vi "Sysdef.SimpleImport.vi"(7 "Overwrite Existing?":bool=TRUE, 8 "error in (no error)":errorcluster, 10 "SysDef":T1 {"Tree"."Properties"."Type" items=["K_STRING", "K_BOOL", "K_I32", "K_U32", "K_DOUBLE", "K_U64", "K_VARIANT", "K_DEPENDENTFILE", "K_DEPENDENTNODE", "K_DATASOURCENODE", "K_U16", "K_DBLARR", "K_U32ARR", "K_I32ARR", "K_STRINGARR", "K_DICTIONARY", "K_DICTIONARYARR"]}, 11 "NodeID":u64) -> (0 "error out":errorcluster, 3 "NodeID out":u64)   [LabVIEW 2015, in "Import - Export CD Config Utility.lvlib"]
doc: "Uses the NI VeriStand .NET API. to add or edit the Custom Device Hierarchy (Sections, Channels, Waveforms) as well as its Items Properties using the data from the SysDef cluster."
uses:
  Import - Export CD Config Utility.lvlib
  _Types/SysDef.Export.ctl
  _Types/TreeItem.ctl
  _Types/TreeItem.Info.ctl
  <vilib>/NI Veristand/Custom Device API/Custom Device Channel.ctl
  <vilib>/NI Veristand/Custom Device API/Custom Device Channel Type.ctl
  <vilib>/NI Veristand/Custom Device API/Custom Device Waveform.ctl
  <vilib>/NI Veristand/Custom Device API/Custom Device Waveform DataType.ctl
  _Types/TreeItem.Property.ctl
  NationalInstruments.VeriStand.SystemDefinitionAPI
  NationalInstruments.VeriStand.SystemStorage
  <vilib>/NI Veristand/Custom Device API/Custom Device API.lvlib
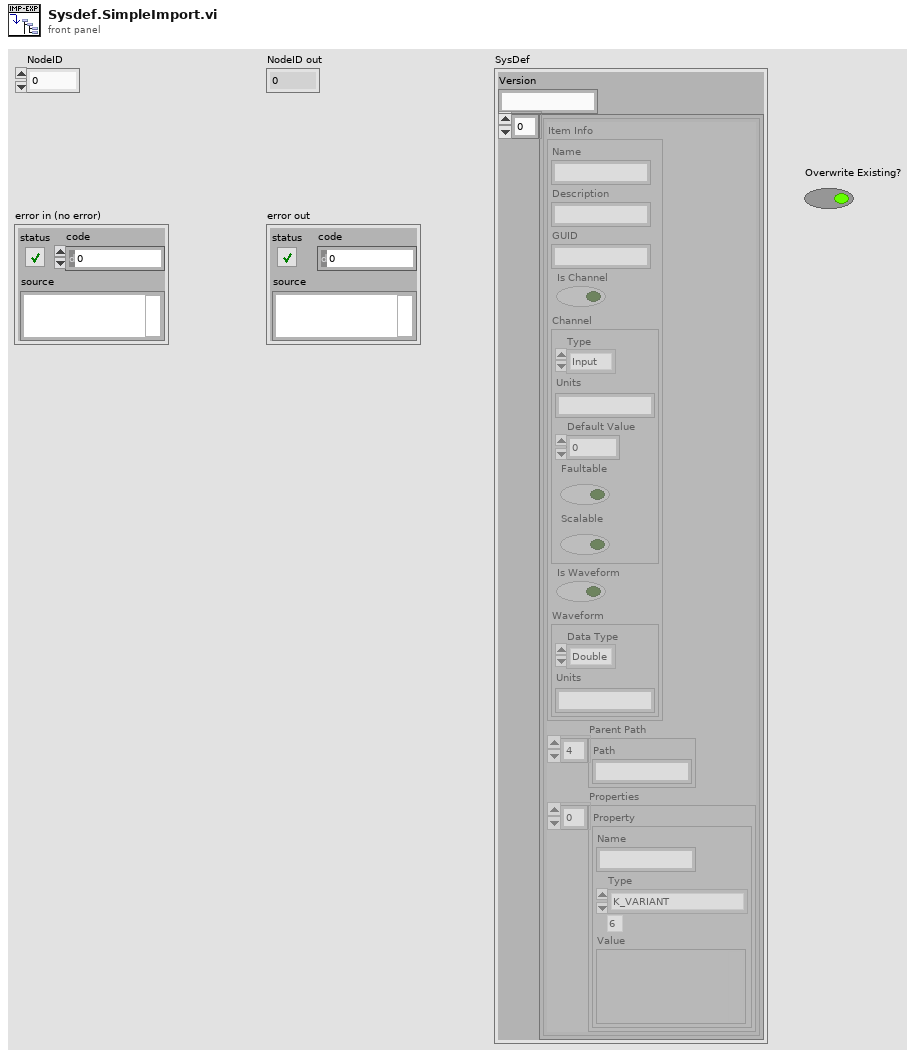
[diagram p1: front panel]
types:
  T1 = typedef "Import - Export CD Config Utility.lvlib/SysDef.Export.ctl" = cluster{"Version":string, "Tree":T2[]}
  T2 = typedef "Import - Export CD Config Utility.lvlib/TreeItem.ctl" = cluster{"Item Info":T3, "Parent Path":string[], "Properties":T8[]}
  T3 = typedef "Import - Export CD Config Utility.lvlib/TreeItem.Info.ctl" = cluster{"Name":string, "Description":string, "GUID":string, "Is Channel":bool, "Channel":T4, "Is Waveform":bool, "Waveform":T6}
  T4 = typedef "Custom Device API.lvlib/Custom Device Channel.ctl" = cluster{"Type":T5, "Units":string, "Default Value":dbl, "Faultable":bool, "Scalable":bool}
  T5 = typedef "Custom Device API.lvlib/Custom Device Channel Type.ctl" = enum16{"Input", "Output"}
  T6 = typedef "Custom Device API.lvlib/Custom Device Waveform.ctl" = cluster{"Data Type":T7, "Units":string}
  T7 = typedef "Custom Device API.lvlib/Custom Device Waveform DataType.ctl" = enum16{"Double", "Complex Double"}
  T8 = typedef "Import - Export CD Config Utility.lvlib/TreeItem.Property.ctl" = cluster{"Name":string, "Type":i32, "Value":variant}
  T9 = typedef "Custom Device API.lvlib/Custom Device Item Ref.ctl" = u64
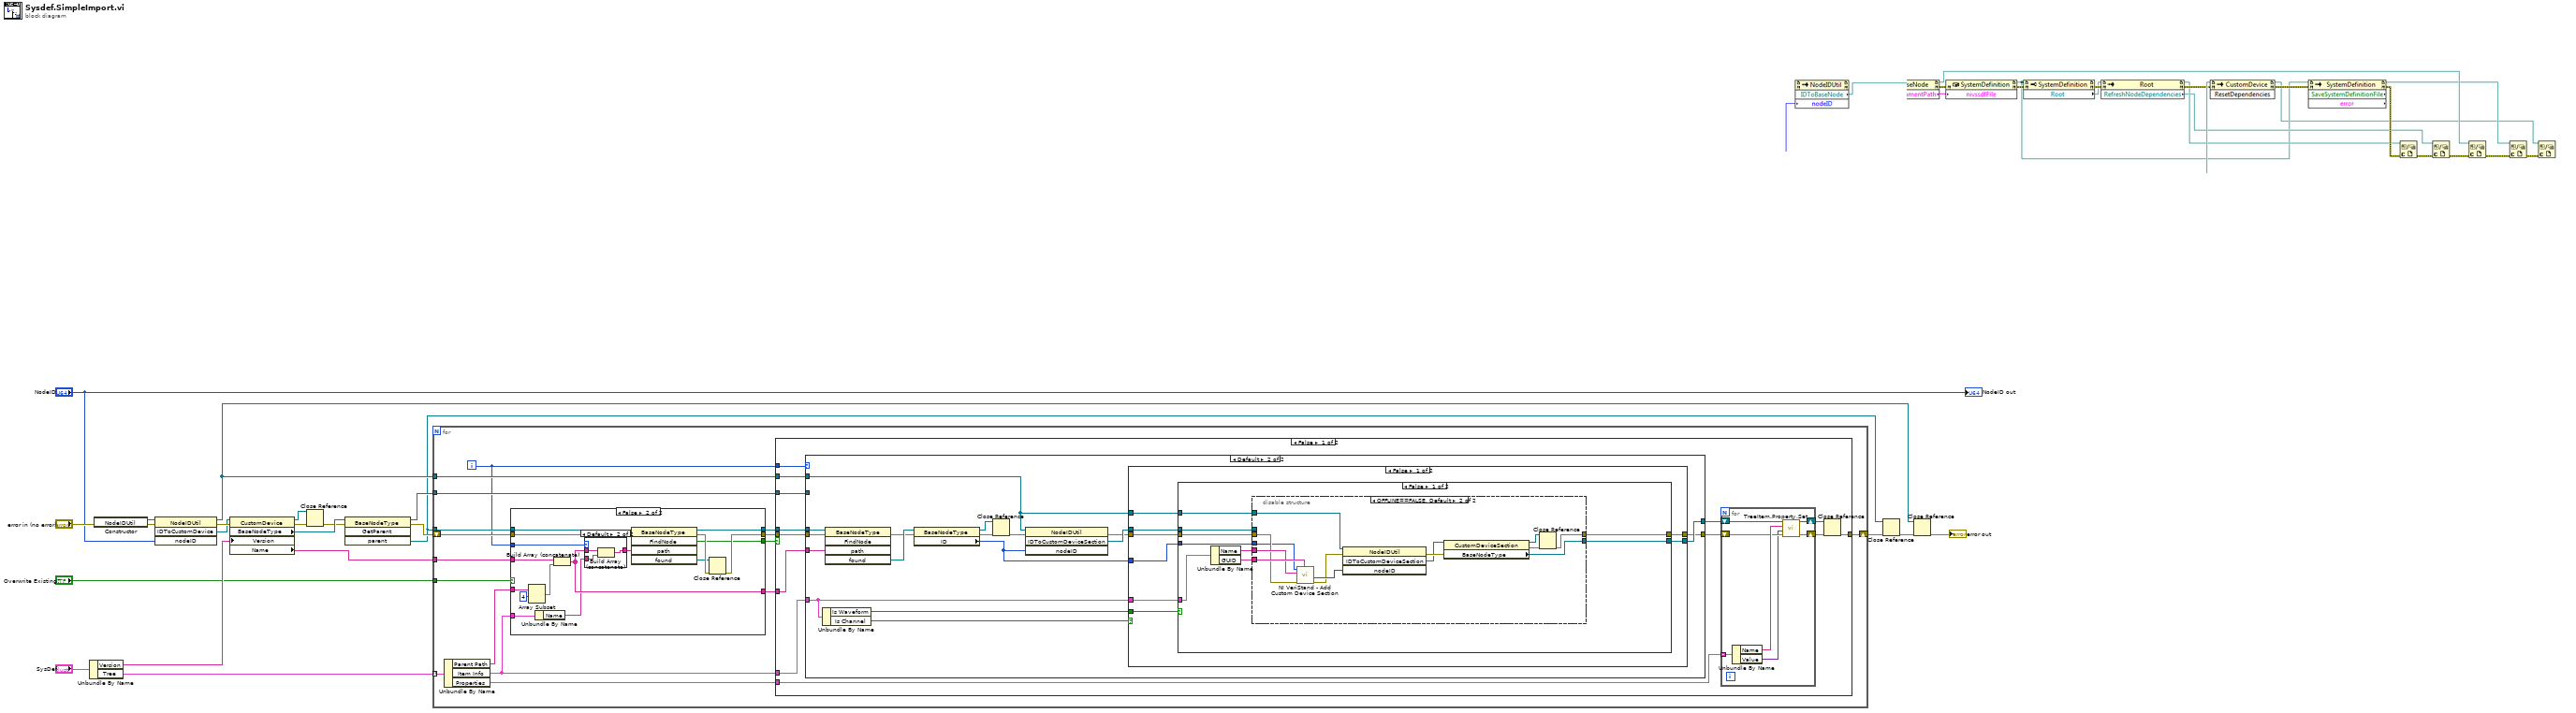
[diagram p0: block diagram]
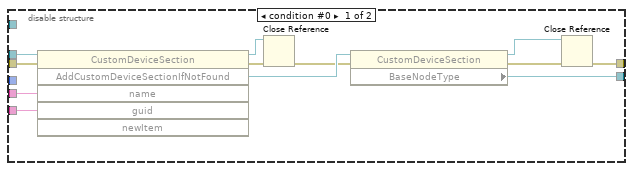
[diagram p3: hidden frame]
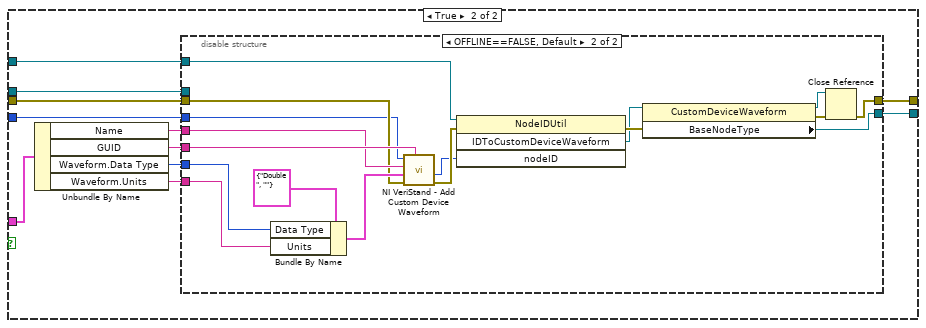
[diagram p4: hidden frame]
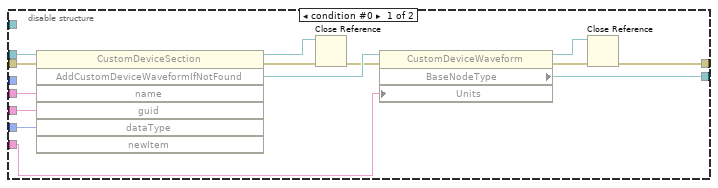
[diagram p5: hidden frame]
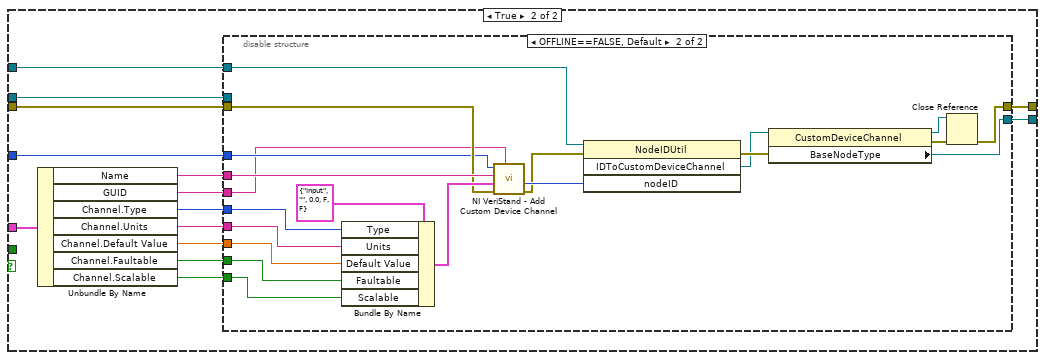
[diagram p6: hidden frame]
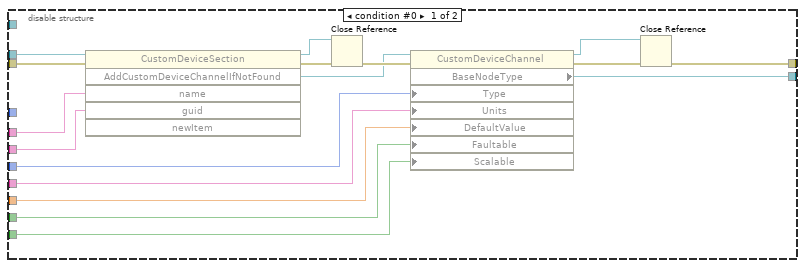
[diagram p7: hidden frame]
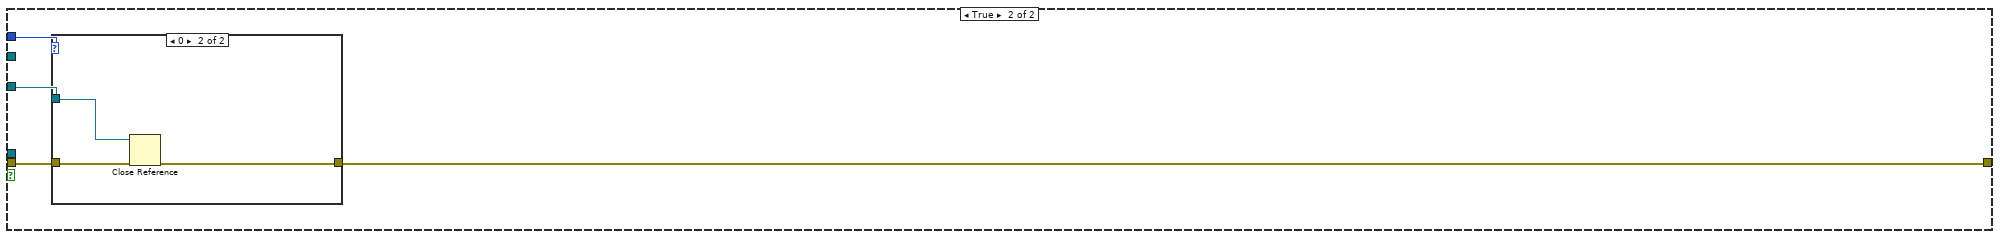
[diagram p8: hidden frame]
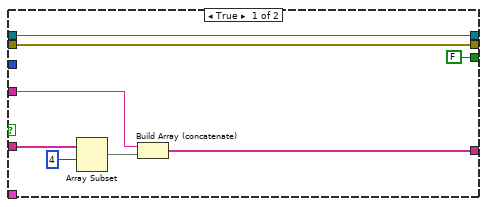
[diagram p10: hidden frame]
diagram:
  n1 = Unbundle By Name("SysDef") -> ("Version"=w20:string, "Tree"=w21:T2[])
  n2 = constructor class="NodeIDUtil"(error in="error in (no error)") -> (reference out=w2:refnum<k24>, error out=w7:errorcluster)  [unwired: 2 in, 1 out]
  n3 = invoke class="NodeIDUtil" method="IDToCustomDevice"(reference=w2, error in=w7, "nodeID"="NodeID") -> (reference out=w13:refnum<k24>, error out=w19:errorcluster, "IDToCustomDevice"=w1:refnum<k24>)  [unwired: 1 in, 1 out]
  n4 = property class="CustomDevice"(reference=w1, error in=w19, "Version"=w20) -> (reference out=w5:refnum<k24>, error out=w4:errorcluster, "BaseNodeType"=w10:refnum<k24>, "Name"=w16:string)
  n5 = Close Reference(reference=w5, error in (no error)=w4) -> (error out=w3:errorcluster)
  n6 = invoke class="BaseNodeType" method="GetParent"(reference=w10, error in=w3) -> (reference out=w17:refnum<k24>, error out=w18:errorcluster, "parent"=w9:refnum<k24>)  [unwired: 2 in, 1 out]
  n7 = for {
    tunnel: w21 -> [w38] mode=indexing
    shift-right: [w35] -> w6
    shift-left: w18 -> [w29]
    tunnel: w17 -> [w34]
    tunnel: w16 -> [w33]
    tunnel: "Overwrite Existing?" -> [w30]
    tunnel: w13 -> [w25]
    tunnel: w9 -> [w24]
    i -> [w23]
    n8 = Unbundle By Name(w38) -> ("Parent Path"=w36:string[], "Item Info"=w31:T3, "Properties"=w37:T8[])
    n9 = case shown="False" w30 {
      tunnel: w36 -> [w227 w243]
      tunnel: w33 -> [w225 w241]
      tunnel: [w224 w239] -> w32
      tunnel: w31 -> [_ w240]
      tunnel: w29 -> [w222 w237]
      tunnel: w24 -> [w223 w235]
      tunnel: [w223 w229] -> w28
      tunnel: [w222 w233] -> w27
      tunnel: [FALSE ("FindNode") w232] -> w26
      tunnel: w23 -> [_ w231]
      frame True {
        n10 = Array Subset(array=w227, index=4) -> (w226:string[])  [unwired: 1 in]
        n11 = Build Array (concatenate)(w225, w226) -> (w224:string[])
      }
      frame False {
        n12 = Array Subset(array=w243, index=4) -> (w242:string[])  [unwired: 1 in]
        n13 = Unbundle By Name(w240) -> ("Name"=w238:string)
        n14 = Build Array (concatenate)(w241, w242) -> (w239:string[])
        n15 = case shown="Default" w231 {
          tunnel: w239 -> [w245 w248]
          tunnel: w238 -> [_ w247]
          tunnel: [w245 w246] -> w236
          frame 0 {
          }
          frame Default {
            n16 = Build Array (concatenate)(w248, w247) -> (w246:string[])
          }
        }
        n17 = invoke class="BaseNodeType" method="FindNode"(reference=w235, error in=w237, "path"=w236) -> (reference out=w229:refnum<k24>, error out=w234:errorcluster, "FindNode"=w232:bool, "found"=w230:refnum<k24>)  [unwired: 2 in, 1 out]
        n18 = Close Reference(reference=w230, error in (no error)=w234) -> (error out=w233:errorcluster)
      }
    }
    n19 = case shown="False" w26 {
      tunnel: w37 -> [w50 _]
      tunnel: w25 -> [w48 _]
      tunnel: [w45 w213] -> w35
      tunnel: w23 -> [w44 w216]
      tunnel: w34 -> [w43 w214]
      tunnel: w32 -> [w42 _]
      tunnel: w31 -> [w41 _]
      tunnel: w28 -> [w40 _]
      tunnel: w27 -> [w39 w215]
      frame False {
        n20 = case shown="Default" w44 {
          tunnel: w39 -> [w52 w68]
          tunnel: [w52 w60] -> w51
          tunnel: [w53 w61] -> w49
          tunnel: w40 -> [_ w56]
          tunnel: w42 -> [_ w70]
          tunnel: w41 -> [_ w62]
          tunnel: w48 -> [_ w54]
          tunnel: w43 -> [w53 _]
          frame 0 {
          }
          frame Default {
            n21 = Unbundle By Name(w62) -> ("Is Waveform"=w59:bool, "Is Channel"=w63:bool)
            n22 = invoke class="BaseNodeType" method="FindNode"(reference=w56, error in=w68, "path"=w70) -> (error out=w67:errorcluster, "found"=w69:refnum<k24>)  [unwired: 2 in, 3 out]
            n23 = property class="BaseNodeType"(reference=w69, error in=w67) -> (reference out=w57:refnum<k24>, error out=w66:errorcluster, "ID"=w55:u64)
            n24 = Close Reference(reference=w57, error in (no error)=w66) -> (error out=w58:errorcluster)
            n25 = invoke class="NodeIDUtil" method="IDToCustomDeviceSection"(reference=w54, error in=w58, "nodeID"=w55) -> (error out=w64:errorcluster, "IDToCustomDeviceSection"=w65:refnum<k24>)  [unwired: 1 in, 2 out]
            n26 = case shown="False" w63 {
              tunnel: w65 -> [w77 w164]
              tunnel: w64 -> [w76 w161]
              tunnel: w62 -> [w74 w157]
              tunnel: [w75 w160] -> w61
              tunnel: [w73 w158] -> w60
              tunnel: w59 -> [w78 _]
              tunnel: w55 -> [w72 w156]
              tunnel: w54 -> [w71 w155]
              frame False {
                n27 = case shown="False" w78 {
                  tunnel: w77 -> [w86 w123]
                  tunnel: w76 -> [w87 w122]
                  tunnel: [w83 w116] -> w75
                  tunnel: [w82 w118] -> w73
                  tunnel: w74 -> [w85 w121]
                  tunnel: w72 -> [w80 w114]
                  tunnel: w71 -> [w79 w113]
                  frame False {
                    n28 = Unbundle By Name(w85) -> ("Name"=w81:string, "GUID"=w84:string)
                    n29 = disable-structure shown="OFFLINE==FALSE, Default" {
                      disable-tunnel: w87 -> [w97 w110]
                      disable-tunnel: w86 -> [w96 _]
                      disable-tunnel: w84 -> [w95 w112]
                      disable-tunnel: [w93 w101] -> w83
                      disable-tunnel: [w89 w100] -> w82
                      disable-tunnel: w81 -> [w88 w111]
                      disable-tunnel: w80 -> [_ w109]
                      disable-tunnel: w79 -> [_ w102]
                      frame condition #0 {
                        n30 = invoke class="CustomDeviceSection" method="AddCustomDeviceSectionIfNotFound"(reference=w96, error in=w97, "name"=w88, "guid"=w95) -> (reference out=w98:refnum<k24>, error out=w99:errorcluster, "AddCustomDeviceSectionIfNotFound"=w94:refnum<k24>)  [unwired: 2 in, 3 out]
                        n31 = Close Reference(reference=w98, error in (no error)=w99) -> (error out=w92:errorcluster)
                        n32 = property class="CustomDeviceSection"(reference=w94, error in=w92) -> (reference out=w91:refnum<k24>, error out=w90:errorcluster, "BaseNodeType"=w93:refnum<k24>)
                        n33 = Close Reference(reference=w91, error in (no error)=w90) -> (error out=w89:errorcluster)
                      }
                      frame condition #1 (active) {
                        n34 = call <vilib>:"NI VeriStand - Add Custom Device Section.vi"("GUID (Default Section)"=w112, "error in (no error)"=w110, "Section Name"=w111, "Parent Ref in"=w109) -> ("error out"=w103:errorcluster, "Section Ptr"=w104:T9)  [unwired: 4 in, 2 out]
                        n35 = invoke class="NodeIDUtil" method="IDToCustomDeviceSection"(reference=w102, error in=w103, "nodeID"=w104) -> (error out=w108:errorcluster, "IDToCustomDeviceSection"=w107:refnum<k24>)  [unwired: 1 in, 2 out]
                        n36 = property class="CustomDeviceSection"(reference=w107, error in=w108) -> (reference out=w106:refnum<k24>, error out=w105:errorcluster, "BaseNodeType"=w101:refnum<k24>)
                        n37 = Close Reference(reference=w106, error in (no error)=w105) -> (error out=w100:errorcluster)
                      }
                    }
                  }
                  frame True {
                    n38 = Unbundle By Name(w121) -> ("Name"=w115:string, "GUID"=w120:string, "Waveform.Data Type"=w119:T7, "Waveform.Units"=w117:string)
                    n39 = disable-structure shown="OFFLINE==FALSE, Default" {
                      disable-tunnel: w123 -> [w133 _]
                      disable-tunnel: w122 -> [w132 w148]
                      disable-tunnel: w120 -> [w131 w154]
                      disable-tunnel: w119 -> [w130 w152]
                      disable-tunnel: [w127 w142] -> w118
                      disable-tunnel: w117 -> [w126 w151]
                      disable-tunnel: [w125 w141] -> w116
                      disable-tunnel: w115 -> [w124 w149]
                      disable-tunnel: w114 -> [_ w139]
                      disable-tunnel: w113 -> [_ w138]
                      frame condition #0 {
                        n40 = invoke class="CustomDeviceSection" method="AddCustomDeviceWaveformIfNotFound"(reference=w133, error in=w132, "name"=w124, "guid"=w131, "dataType"=w130) -> (reference out=w136:refnum<k24>, error out=w137:errorcluster, "AddCustomDeviceWaveformIfNotFound"=w135:refnum<k24>)  [unwired: 2 in, 4 out]
                        n41 = Close Reference(reference=w136, error in (no error)=w137) -> (error out=w134:errorcluster)
                        n42 = property class="CustomDeviceWaveform"(reference=w135, error in=w134, "Units"=w126) -> (reference out=w129:refnum<k24>, error out=w128:errorcluster, "BaseNodeType"=w125:refnum<k24>)
                        n43 = Close Reference(reference=w129, error in (no error)=w128) -> (error out=w127:errorcluster)
                      }
                      frame condition #1 (active) {
                        n44 = Bundle By Name(cluster=T6 {"Data Type"=enum."Double", "Units"=""} ("Waveform"), "Data Type"=w152, "Units"=w151) -> (w150:T6)
                        n45 = call <vilib>:"NI VeriStand - Add Custom Device Waveform.vi"("GUID (Default Waveform)"=w154, "error in (no error)"=w148, "Waveform"=w150, "Waveform Name"=w149, "Parent Ref in"=w139) -> ("error out"=w143:errorcluster, "Waveform Ref"=w140:T9)  [unwired: 3 in, 2 out]
                        n46 = invoke class="NodeIDUtil" method="IDToCustomDeviceWaveform"(reference=w138, error in=w143, "nodeID"=w140) -> (error out=w147:errorcluster, "IDToCustomDeviceWaveform"=w146:refnum<k24>)  [unwired: 1 in, 2 out]
                        n47 = property class="CustomDeviceWaveform"(reference=w146, error in=w147) -> (reference out=w145:refnum<k24>, error out=w144:errorcluster, "BaseNodeType"=w141:refnum<k24>)
                        n48 = Close Reference(reference=w145, error in (no error)=w144) -> (error out=w142:errorcluster)
                      }
                    }
                  }
                }
              }
              frame True {
                n49 = Unbundle By Name(w157) -> ("Name"=w159:string, "GUID"=w163:string, "Channel.Type"=w162:T5, "Channel.Units"=w168:string, "Channel.Default Value"=w167:dbl, "Channel.Faultable"=w166:bool, "Channel.Scalable"=w165:bool)
                n50 = disable-structure shown="OFFLINE==FALSE, Default" {
                  disable-tunnel: w168 -> [w184 w202]
                  disable-tunnel: w167 -> [w183 w201]
                  disable-tunnel: w166 -> [w182 w200]
                  disable-tunnel: w165 -> [w181 w199]
                  disable-tunnel: w164 -> [w180 _]
                  disable-tunnel: w163 -> [w179 w186]
                  disable-tunnel: w162 -> [w178 w203]
                  disable-tunnel: w161 -> [w176 w197]
                  disable-tunnel: [w175 w193] -> w160
                  disable-tunnel: w159 -> [w174 w205]
                  disable-tunnel: [w173 w187] -> w158
                  disable-tunnel: w156 -> [_ w196]
                  disable-tunnel: w155 -> [_ w194]
                  frame condition #0 {
                    n51 = invoke class="CustomDeviceSection" method="AddCustomDeviceChannelIfNotFound"(reference=w180, error in=w176, "name"=w174, "guid"=w179) -> (reference out=w169:refnum<k24>, error out=w172:errorcluster, "AddCustomDeviceChannelIfNotFound"=w170:refnum<k24>)  [unwired: 2 in, 3 out]
                    n52 = Close Reference(reference=w169, error in (no error)=w172) -> (error out=w185:errorcluster)
                    n53 = property class="CustomDeviceChannel"(reference=w170, error in=w185, "Type"=w178, "Units"=w184, "DefaultValue"=w183, "Faultable"=w182, "Scalable"=w181) -> (reference out=w177:refnum<k24>, error out=w171:errorcluster, "BaseNodeType"=w175:refnum<k24>)
                    n54 = Close Reference(reference=w177, error in (no error)=w171) -> (error out=w173:errorcluster)
                  }
                  frame condition #1 (active) {
                    n55 = Bundle By Name(cluster=T4 {"Type"=enum."Input", "Units"="", "Default Value"=0.0, "Faultable"=FALSE, "Scalable"=FALSE} ("Channel"), "Type"=w203, "Units"=w202, "Default Value"=w201, "Faultable"=w200, "Scalable"=w199) -> (w198:T4)
                    n56 = call <vilib>:"NI VeriStand - Add Custom Device Channel.vi"("GUID (Default Channel)"=w186, "error in (no error)"=w197, "Channel"=w198, "Channel Name"=w205, "Parent Ref in"=w196) -> ("error out"=w192:errorcluster, "Channel Ref"=w195:T9)  [unwired: 3 in, 2 out]
                    n57 = invoke class="NodeIDUtil" method="IDToCustomDeviceChannel"(reference=w194, error in=w192, "nodeID"=w195) -> (error out=w191:errorcluster, "IDToCustomDeviceChannel"=w190:refnum<k24>)  [unwired: 1 in, 2 out]
                    n58 = property class="CustomDeviceChannel"(reference=w190, error in=w191) -> (reference out=w189:refnum<k24>, error out=w188:errorcluster, "BaseNodeType"=w193:refnum<k24>)
                    n59 = Close Reference(reference=w189, error in (no error)=w188) -> (error out=w187:errorcluster)
                  }
                }
              }
            }
          }
        }
        n60 = for {
          shift-right: [w212] -> w46
          shift-left: w51 -> [w207]
          tunnel: w50 -> [w210] mode=indexing
          shift-right: [w209] -> w47
          shift-left: w49 -> [w211]
          n61 = Unbundle By Name(w210) -> ("Name"=w208:string, "Value"=w206:variant)
          n62 = call "TreeItem.Property.Set.vi"("error in (no error)"=w207, "Value"=w206, "Property Name"=w208, "BaseNodeType"=w211) -> ("error out"=w212:errorcluster, "BaseNodeType"=w209:refnum<k24>)  [unwired: 5 in, 1 out]
        }
        n63 = Close Reference(reference=w47, error in (no error)=w46) -> (error out=w45:errorcluster)
      }
      frame True {
        n64 = case shown="0" w216 {
          tunnel: w215 -> [w217 w220]
          tunnel: [w217 w219] -> w213
          tunnel: w214 -> [_ w218]
          frame Default {
          }
          frame 0 {
            n65 = Close Reference(reference=w218, error in (no error)=w220) -> (error out=w219:errorcluster)
          }
        }
      }
    }
  }
  n66 = Close Reference(reference=w9, error in (no error)=w6) -> (error out=w14:errorcluster)
  n67 = Close Reference(reference=w13, error in (no error)=w14) -> (error out=→"error out":errorcluster)
  "NodeID out" <- "NodeID"
